vi "FilePathFGV.vi"(0 "selected path":path caption="Ubicación archivo IN", 4 "Opción":enum16{"Write", "Read"}(ring), 5 "Error In":errorcluster) -> (14 "selected path 2":path caption="Ubicación archivo OUT", 19 "Error Out":errorcluster)   [LabVIEW 2013]
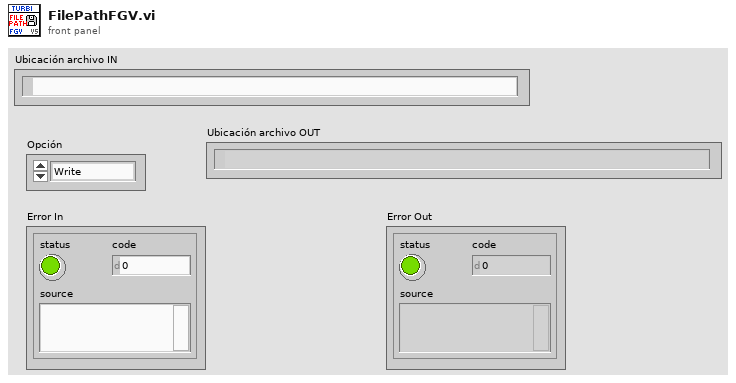
[diagram p1: front panel]
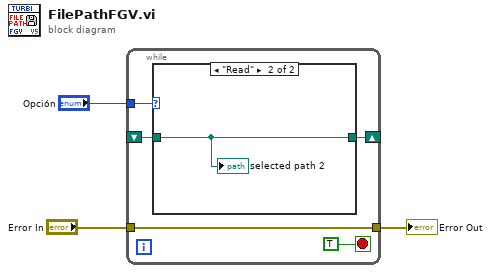
[diagram p0: block diagram]
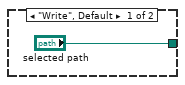
[diagram p2: hidden frame]
diagram:
  n1 = while {
    tunnel: "Opción" -> [w7]
    tunnel: [w6] -> w2
    tunnel: "Error In" -> [w6]
    shift-right: [w5] -> _
    shift-left: _ -> [w4]
    stop <- TRUE stop-if-true
    n2 = case shown="\"Read\"" w7 {
      tunnel: ["selected path" w10] -> w5
      tunnel: w4 -> [_ w10]
      frame "Write", Default {
      }
      frame "Read" {
        "selected path 2" <- w10
      }
    }
  }
  "Error Out" <- w2
